vi "Reference Path.vi"(11 "a,b":dbl[](array[numeric])) -> (3 "Circular Path":cluster{dbl[], dbl[]})   [LabVIEW 2021]
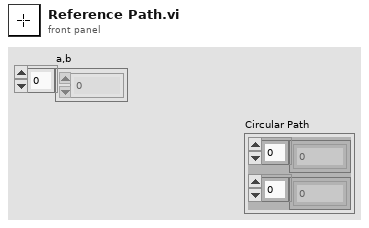
[diagram p1: front panel]
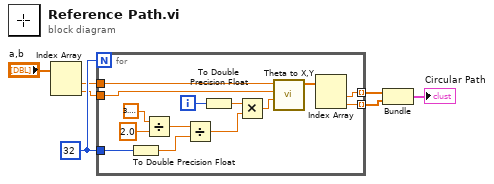
[diagram p0: block diagram]
diagram:
  w6 = 32 ("Drawing Samples")
  n1 = Index Array(array="a,b") -> (element #1=w3:dbl, element #2=w1:dbl)  [unwired: 2 in]
  n2 = for {
    N: w6 -> [_]
    tunnel: [w9] -> w4 mode=indexing
    tunnel: [w8] -> w5 mode=indexing
    tunnel: w6 -> [w19]
    tunnel: w3 -> [w12]
    tunnel: w1 -> [w11]
    i -> [w20]
    n3 = To Double Precision Float(number=w19) -> (double precision float=w17:dbl)
    n4 = Divide(x=3.141592653589793, y=2.0 ("x")) -> (x/y=w16:dbl)
    n5 = Divide(x=w16, y=w17) -> (x/y=w21:dbl)
    n6 = To Double Precision Float(number=w20) -> (double precision float=w18:dbl)
    n7 = Multiply(x=w18, y=w21) -> (x*y=w13:dbl)
    n8 = call "Theta to X,Y.vi"("theta"=w13, "b"=w11, "a"=w12) -> ("X,Y"=w10:dbl[])  [unwired: 8 in]
    n9 = Index Array(array=w10) -> (element #1=w9:dbl, element #2=w8:dbl)  [unwired: 2 in]
  }
  n10 = Bundle(w4, w5) -> (→"Circular Path":cluster{dbl[], dbl[]})  [unwired: 1 in]
